vi "UMLEditor GetClassAttributeFile.vi"(2 "ClassName":string, 3 "ClassPath":path) -> (0 "Ctrl-File":bool, 1 "AttributePath":path)   [LabVIEW 2014]
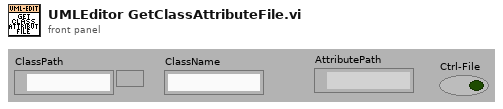
[diagram p1: front panel]
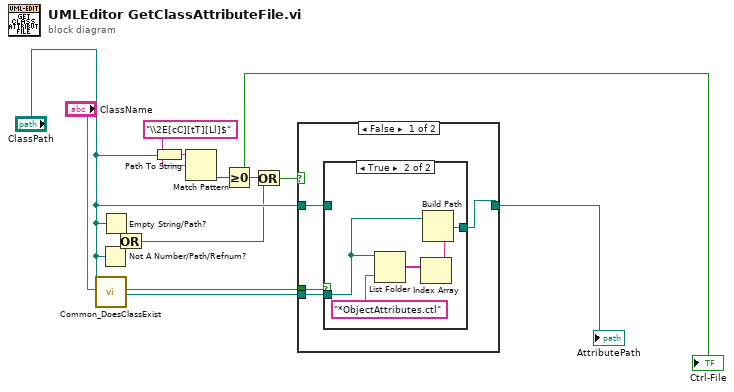
[diagram p0: block diagram]
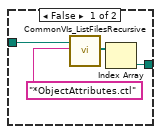
[diagram p2: hidden frame]
diagram:
  n1 = call <resource>:"Common_DoesClassExist.vi"("ClassPath"="ClassPath", "ClassName"="ClassName") -> ("llb-class"=w12:bool, "llb/LvCLass-Path"=w13:path)  [unwired: 16 out]
  n2 = Not A Number/Path/Refnum?(number/path/refnum="ClassPath") -> (NaN/Path/Refnum?=w4:bool)
  n3 = Empty String/Path?(string/path="ClassPath") -> (empty?=w5:bool)
  n4 = Or(x=w5, y=w4) -> (x .or. y?=w7:bool)
  n5 = Path To String(path="ClassPath") -> (string=w2:string)
  n6 = Match Pattern(string=w2, regular expression="\\2E[cC][tT][Ll]$") -> (offset past match=w3:i32)  [unwired: 4 out]
  n7 = Greater Or Equal To 0?(x=w3) -> (x >= 0?=w9:bool)
  "Ctrl-File" <- w9
  n8 = Or(x=w9, y=w7) -> (x .or. y?=w6:bool)
  n9 = case shown="False" w6 {
    tunnel: "ClassPath" -> [w17 w27]
    tunnel: [w16 w27] -> w8
    tunnel: w12 -> [w15 _]
    tunnel: w13 -> [w14 _]
    frame False {
      n10 = case shown="True" w15 {
        tunnel: w17 -> [w21 _]
        tunnel: [w18 w22] -> w16
        tunnel: w14 -> [_ w25]
        frame False {
          n11 = call <resource>:"CommonVIs_ListFilesRecursive.vi"("directory path"=w21, "FileSearchPattern"="*ObjectAttributes.ctl") -> ("Files"=w19:path[])  [unwired: 4 in, 13 out]
          n12 = Index Array(array=w19) -> (element=w18:path)  [unwired: 1 in]
        }
        frame True {
          n13 = List Folder(path=w25, pattern="*ObjectAttributes.ctl" ("FileSearchPattern")) -> (filenames=w24:string[])  [unwired: 1 in, 4 out]
          n14 = Index Array(array=w24) -> (element=w23:string)  [unwired: 1 in]
          n15 = Build Path(base path=w25, name or relative path=w23) -> (appended path=w22:path)
        }
      }
    }
    frame True {
    }
  }
  "AttributePath" <- w8
